vi "Create Laser Process.vi"(8 "error in (no error)":errorcluster, 10 "Laser Driver.lvclass":refnum<class "Laser Driver.lvclass">, 11 "Laser Controller in":refnum<class "Laser Controller.lvclass">) -> (0 "error out":errorcluster, 3 "Laser Controller":refnum<class "Laser Controller.lvclass">)   [LabVIEW 2022 SP3, in "Laser Process.lvlib" / "Laser Process.lvclass"]
uses:
  Laser Process.lvclass
  Laser Process.lvclass/Laser Process.ctl
  XY Stage/Process Actor/Process Framework/Process State Data/Process State Data.lvclass
  XY Stage/Process Actor/Process Framework/Interlock Q Class/Interlock Q Class.lvclass
  <vilib>/ActorFramework/Actor/Actor.lvclass
  Laser State Data/Laser State Data.lvclass
  Laser Controller/Laser Controller.lvclass
  C:/Program Files/National Instruments/LabVIEW 2022/vi.lib/MGI/Monitored Actor/Monitored Actor/Monitored Actor/Monitored Actor.lvclass
  C:/Program Files/National Instruments/LabVIEW 2022/vi.lib/ActorFramework/Actor/Actor.lvclass
  C:/XY Stage/Laser/Laser Process/Laser Process/Laser Process.lvclass
  Laser Driver/Laser Driver.lvclass
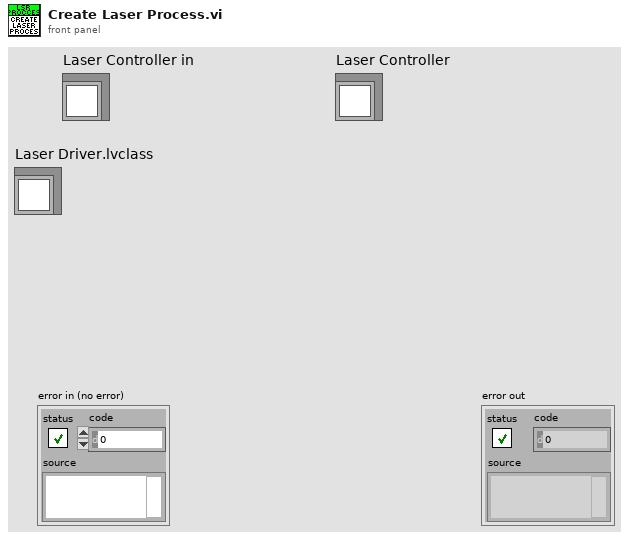
[diagram p1: front panel]
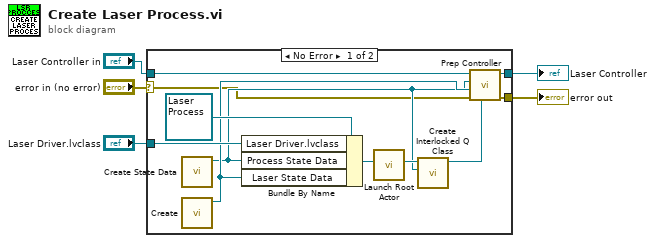
[diagram p0: block diagram]
diagram:
  n1 = case shown="No Error" "error in (no error)" {
    selector: "error in (no error)" -> [w8 w17]
    tunnel: [w7 w17] -> w4
    tunnel: "Laser Driver.lvclass" -> [w15 _]
    tunnel: "Laser Controller in" -> [w12 _]
    tunnel: [w6 _] -> w1
    frame No Error {
      n2 = call "Create State Data.vi"() -> ("Process State Data out"=w10:refnum<data-value>)  [unwired: 10 in, 1 out]
      n3 = call "Create.vi"() -> ("data value reference"=w11:refnum<data-value>)  [unwired: 10 in, 1 out]
      n4 = Bundle By Name(cluster=refnum<class "Laser Process.lvclass"> refnum ("Laser Process.lvlib:Laser Process.lvclass"), "Laser Driver.lvclass"=w15, "Process State Data"=w10, "Laser State Data"=w11) -> (w14:refnum<class "Laser Process.lvclass">)
      n5 = call <vilib>:"Launch Root Actor.vi"("Actor"=w14) -> ("Actor's Enqueuer"=w13:refnum<class "Message Enqueuer.lvclass">)  [unwired: 9 in, 1 out]
      n6 = call "Create Interlocked Q Class.vi"("Process State Data"=w10, "Process Q"=w13) -> ("Interlock Q Class out"=w9:refnum<class "Interlock Q Class.lvclass">)  [unwired: 9 in]
      n7 = call "Prep Controller.vi"("Interlock Q Class out"=w9, "error in (no error)"=w8, "Laser State Data"=w11, "Process State Data"=w10, "Laser Controller in"=w12) -> ("error out"=w7:errorcluster, "Laser Controller out"=w6:refnum<class "Laser Controller.lvclass">)  [unwired: 5 in]
    }
    frame Error {
    }
  }
  "error out" <- w4
  "Laser Controller" <- w1
